vi "PCAN_SPECIAL_Function.vi"(7 "pathCAN_DLL":path, 8 "error in (no error)":errorcluster, 10 "codenumber":i16, 11 "distributorcode":u32) -> (0 "error out":errorcluster, 3 "failed":bool)   [LabVIEW 2023, in "pCANLib.lvlib"]
uses:
  pCANLib.lvlib
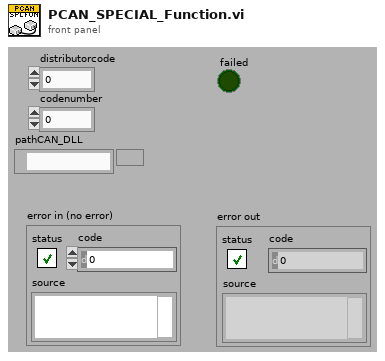
[diagram p1: front panel]
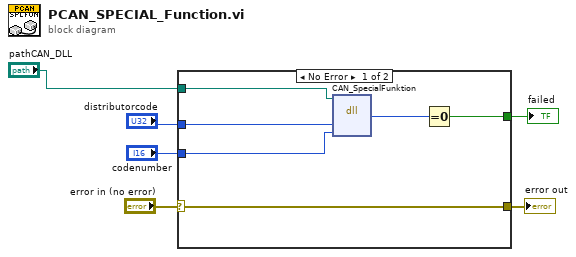
[diagram p0: block diagram]
diagram:
  n1 = case shown="No Error" "error in (no error)" {
    selector: "error in (no error)" -> [w12 w13]
    tunnel: [w12 w13] -> w4
    tunnel: "distributorcode" -> [w11 _]
    tunnel: "codenumber" -> [w10 _]
    tunnel: [w8 _] -> w2
    tunnel: "pathCAN_DLL" -> [w7 _]
    frame No Error {
      n2 = dll-call lib="D:/PCAN/PCAN/PCAN Driver/PCAN_Driver/PCAN_USB.DLL" fn="CAN_SpecialFunktion"(path in=w7, "distributorcode"=w11, "codenumber"=w10) -> ("return type"=w9:i32)  [unwired: 4 in, 2 out]
      n3 = Equal To 0?(x=w9) -> (x = 0?=w8:bool)
    }
    frame Error {
    }
  }
  "error out" <- w4
  "failed" <- w2
